vi "SetSize.vi"(9 "Widht":dbl, 10 "Height":dbl, 11 "TabControl in":refnum<vi>) -> ()   [LabVIEW 2020]
uses:
  <vilib>/Utility/miscctls.llb/LVBoundsTypeDef.ctl
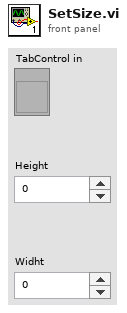
[diagram p1: front panel]
types:
  T1 = typedef "LVBoundsTypeDef.ctl" = cluster{"Width":u32, "Height":u32}
  T2 = typedef "LVPositionTypeDef.ctl" = cluster{"Left":i32, "Top":i32}
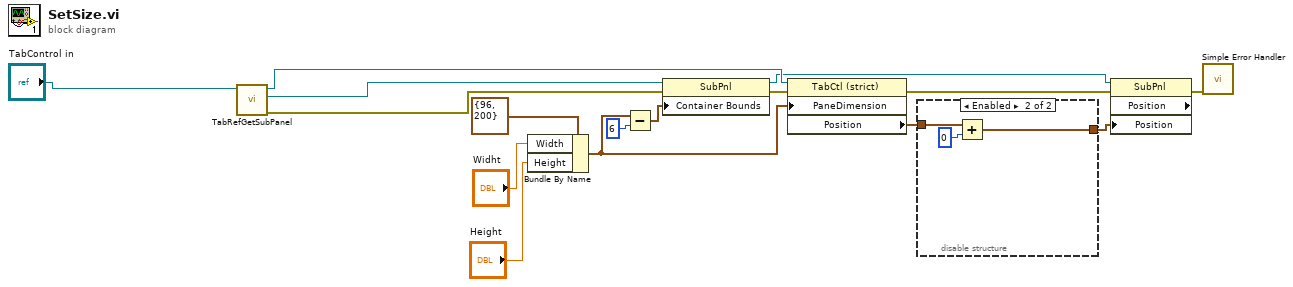
[diagram p0: block diagram]
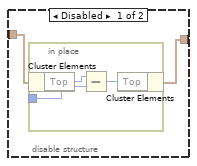
[diagram p2: hidden frame]
diagram:
  n1 = call "TabRefGetSubPanel.vi"("TabControl in"="TabControl in") -> ("error out"=w9:errorcluster, "Sub Panel"=w14:refnum<vi>, "TabControl out"=w16:refnum<vi>)  [unwired: 8 in]
  n2 = Bundle By Name(cluster=T1 {"Width"=96, "Height"=200} ("TabDimension"), "Width"="Widht", "Height"="Height") -> (w1:T1)
  n3 = Subtract(x=w1, y=6) -> (x-y=w2:T1)
  n4 = property class="SubPnl"(reference=w14, error in=w9, "Container Bounds"=w2) -> (reference out=w8:refnum<vi>, error out=w13:errorcluster)
  n5 = property class="TabCtl (strict)"(reference=w16, error in=w13, "PaneDimension"=w1) -> (error out=w7:errorcluster, "Position"=w5:T2)  [unwired: 1 out]
  n6 = disable-structure shown="Enabled" {
    disable-tunnel: w5 -> [w19 w25]
    disable-tunnel: [w18 w23] -> w4
    frame Disabled {
      n7 = in-place {
        in-place-border: [w21] -> w17
        n8 = in-place-cluster #1(w19) -> ("Top"=w22:i32)
        n9 = Subtract(x=w22, y=w21) -> (x-y=w20:i32)
        n10 = in-place-cluster #1("Top"=w20) -> (w18:T2)
      }
    }
    frame Enabled {
      n11 = Add(x=w25, y=0) -> (x+y=w23:T2)
    }
  }
  n12 = property class="SubPnl" props=["Position", "Position"](reference=w8, error in=w7, "Position"=w4) -> (error out=w6:errorcluster)  [unwired: 2 out]
  n13 = call <vilib>:"Simple Error Handler.vi"("error in (no error)"=w6) -> ()  [unwired: 4 in, 5 out]
